vi "Polar Plot - Facade.vi"(0 "Data In":T3 {"phase (deg)" format="%0.2f"; "magnitude" format="%0.2f"}, 2 "Display State In":T1={"Plot Attributes"={"maximum"=2.0, "minimum"=0.0, "clip to min"=FALSE, "log"=FALSE, "grid color"=3381657, "plot color"=16711680, "fmt and prec"={"format"=enum."Decimal", "precision"=2}, "visible section"=4}, "Desired Font"=enum."Application Font", "User-Specified Font"={"Font Name:"="Arial", "Size"=9, "Strikeout?"=FALSE, "Italic?"=FALSE, "Underline?"=FALSE, "Outline?"=FALSE, "Shadow?"=FALSE, "Bold?"=FALSE}} {"Plot Attributes"."minimum" format="%0.2f"; "Plot Attributes"."maximum" format="%0.2f"}, 3 "Container State":T2) -> (6 "Data Out":T3 {"phase (deg)" format="%0.2f"; "magnitude" format="%0.2f"}, 7 "Display State Out":T1={"Plot Attributes"={"maximum"=2.0, "minimum"=0.0, "clip to min"=FALSE, "log"=FALSE, "grid color"=3381657, "plot color"=16711680, "fmt and prec"={"format"=enum."Decimal", "precision"=2}, "visible section"=4}, "Desired Font"=enum."Application Font", "User-Specified Font"={"Font Name:"="Arial", "Size"=9, "Strikeout?"=FALSE, "Italic?"=FALSE, "Underline?"=FALSE, "Outline?"=FALSE, "Shadow?"=FALSE, "Bold?"=FALSE}} {"Plot Attributes"."minimum" format="%0.2f"; "Plot Attributes"."maximum" format="%0.2f"}, 8 "Action":T4)   [LabVIEW 2009, in "Polar Plot.xctl"]
doc: "Demonstration of an XControl.\n\nAAL 9/09"
uses:
  Polar Plot.xctl
  <vilib>/_xctls/Action.ctl
  Polar Plot - Data.ctl
  <vilib>/_xctls/Container State.ctl
  Polar Plot - State.ctl
  <vilib>/_xctls/XControlSupport.lvlib
panel:
  out "Picture":picture
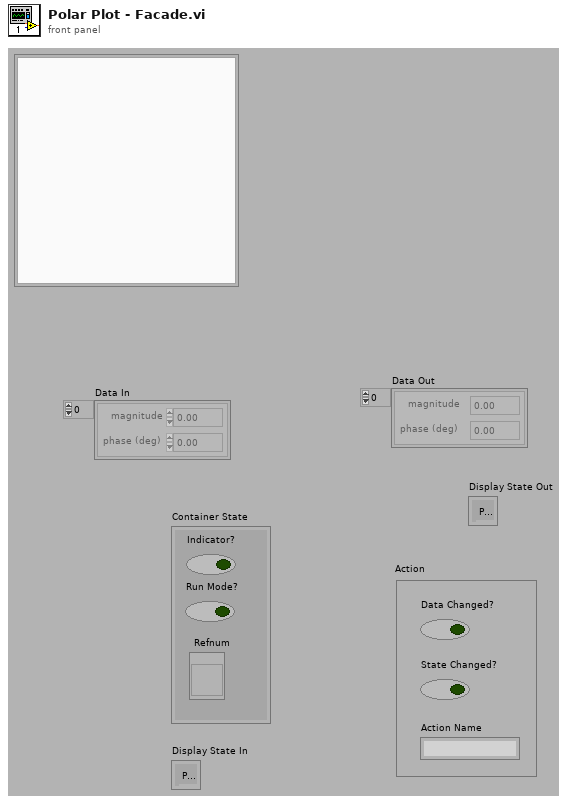
[diagram p1: front panel]
types:
  T1 = typedef "Polar Plot.xctl/Polar Plot - State.ctl" = cluster{"Plot Attributes":cluster{"maximum":dbl, "minimum":dbl, "clip to min":bool, "log":bool, "grid color":u32, "plot color":u32, "fmt and prec":cluster{"format":enum8{"Decimal", "Scientific", "Engineering", "Binary", "Octal", "Hex"}, "precision":u8}, "visible section":u16}, "Desired Font":enum16{"User-specified Font", "Application Font", "System Font", "Dialog Font"}, "User-Specified Font":cluster{"Font Name:":string, "Size":i16, "Strikeout?":bool, "Italic?":bool, "Underline?":bool, "Outline?":bool, "Shadow?":bool, "Bold?":bool}}
  T2 = typedef "XControlSupport.lvlib/Container State.ctl" = cluster{"Indicator?":bool, "Run Mode?":bool, " Refnum":refnum<vi>}
  T3 = typedef "Polar Plot.xctl/Polar Plot - Data.ctl" = cluster{"magnitude":dbl, "phase (deg)":dbl}[]
  T4 = typedef "XControlSupport.lvlib/Action.ctl" = cluster{"Data Changed?":bool, "State Changed?":bool, "Action Name":string}
  T5 = cluster{"Plot Attributes":cluster{"maximum":dbl, "minimum":dbl, "clip to min":bool, "log":bool, "grid color":u32, "plot color":u32, "fmt and prec":cluster{"format":enum8{"Decimal", "Scientific", "Engineering", "Binary", "Octal", "Hex"}, "precision":u8}, "visible section":u16}, "Desired Font":enum16{"User-specified Font", "Application Font", "System Font", "Dialog Font"}, "User-Specified Font":cluster{"Font Name:":string, "Size":i16, "Strikeout?":bool, "Italic?":bool, "Underline?":bool, "Outline?":bool, "Shadow?":bool, "Bold?":bool}}
  T6 = cluster{"Font Name:":string, "Size":i16, "Strikeout?":bool, "Italic?":bool, "Underline?":bool, "Outline?":bool, "Shadow?":bool, "Bold?":bool}
  T7 = enum16{"User-specified Font", "Application Font", "System Font", "Dialog Font"}
  T8 = cluster{"maximum":dbl, "minimum":dbl, "clip to min":bool, "log":bool, "grid color":u32, "plot color":u32, "fmt and prec":cluster{"format":enum8{"Decimal", "Scientific", "Engineering", "Binary", "Octal", "Hex"}, "precision":u8}, "visible section":u16}
  T9 = typedef "LVBoundsTypeDef.ctl" = cluster{"Width":u32, "Height":u32}
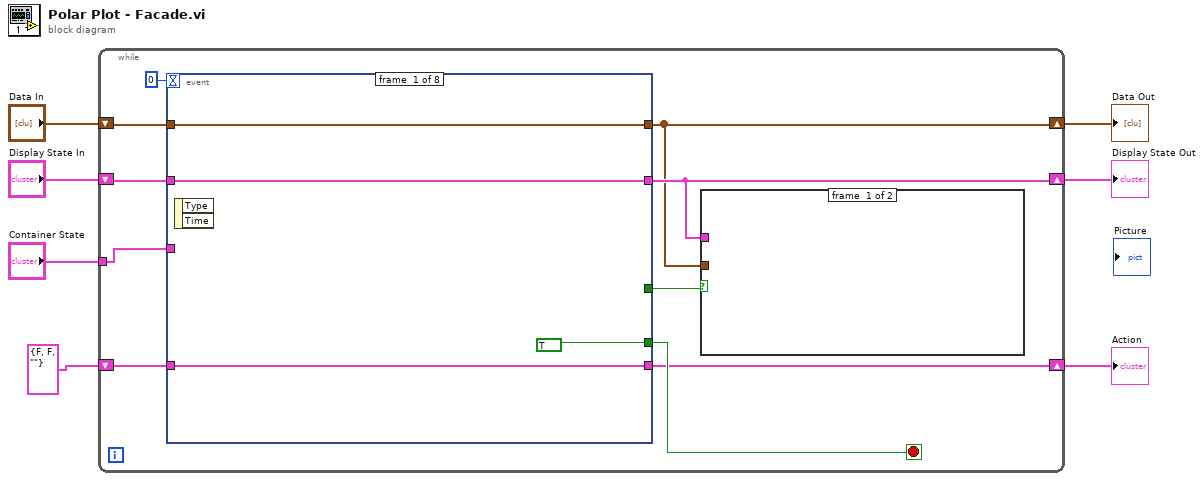
[diagram p0: block diagram]
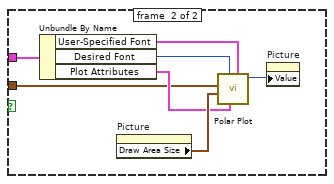
[diagram p2: hidden frame]
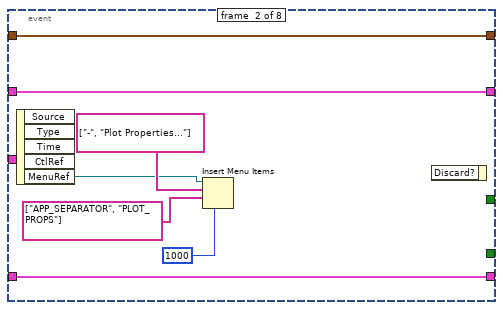
[diagram p3: hidden frame]
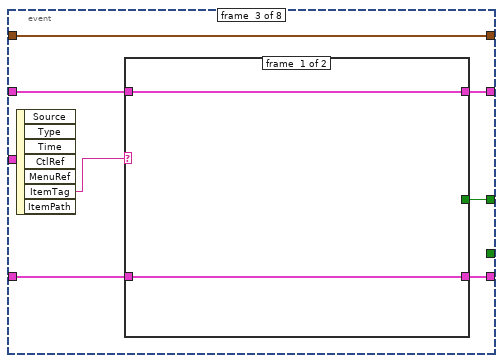
[diagram p4: hidden frame]
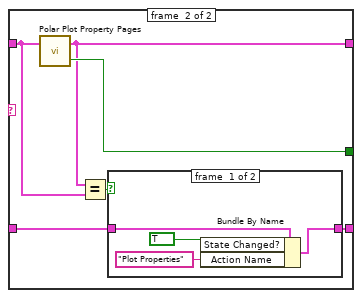
[diagram p5: hidden frame]
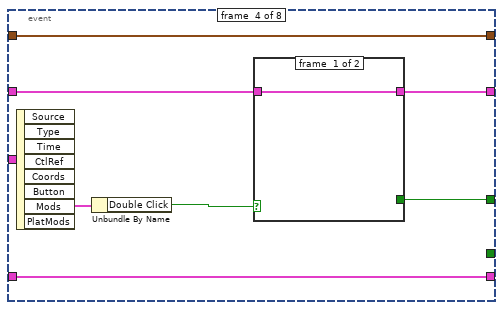
[diagram p7: hidden frame]
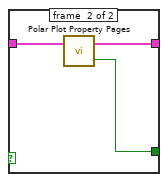
[diagram p8: hidden frame]
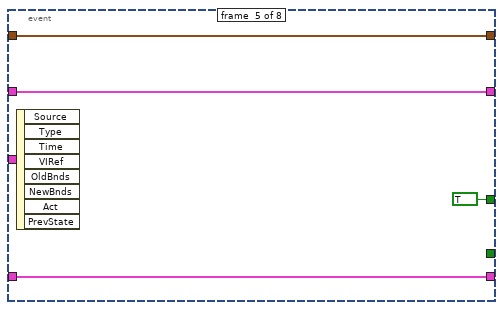
[diagram p9: hidden frame]
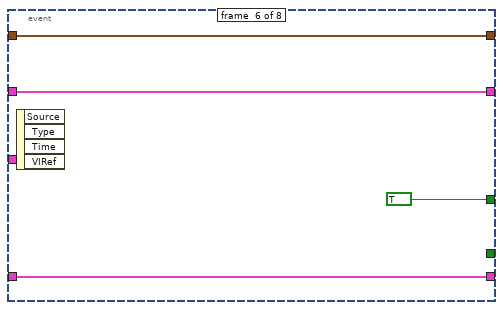
[diagram p10: hidden frame]
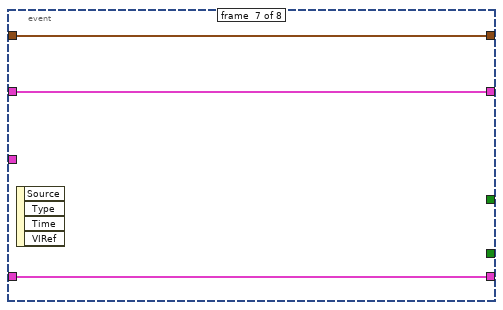
[diagram p11: hidden frame]
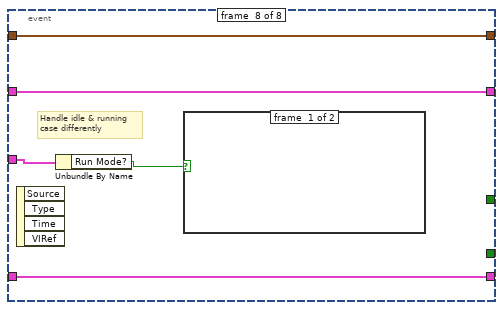
[diagram p12: hidden frame]
diagram:
  n1 = while {
    shift-right: [w9] -> w4
    shift-left: "Display State In" -> [w14]
    tunnel: "Container State" -> [w13]
    shift-right: [w8] -> w7
    shift-left: "Data In" -> [w15]
    shift-right: [w10] -> w1
    shift-left: T4 {"Data Changed?"=FALSE, "State Changed?"=FALSE, "Action Name"=""} ("Data Changed?") -> [w12]
    stop <- w11 stop-if-true
    n2 = event shown="[2] \"Picture\": Shortcut Menu Selection (User)" {
      selector: _ -> [_ _ _ _ _ _ _ _]
      dyn-events: _ -> [_ _ _ _ _ _ _ _]
      timeout: 0 -> [_ _ _ _ _ _ _ _]
      tunnel: w14 -> [w26 w32 w41 w62 w67 w73 w77 w80]
      tunnel: [w26 w32 w40 w61 w67 w73 w77 w80] -> w9
      tunnel: [TRUE _ _ _ _ _ _ _] -> w11
      tunnel: w13 -> [_ _ _ _ _ _ _ w81]
      tunnel: w15 -> [w25 w33 w38 w58 w68 w72 w76 w79]
      tunnel: [w25 w33 w38 w58 w68 w72 w76 w79] -> w8
      tunnel: [w27 w34 w37 w59 w69 w74 w75 w78] -> w10
      tunnel: w12 -> [w27 w34 w36 w59 w69 w74 w75 w78]
      tunnel: [_ _ w39 w60 TRUE ("OK?") TRUE _ _] -> w16
      event #0 {
        n3 = event-data() -> ()  [unwired: 1 in, 2 out]
      }
      event #1 {
        n4 = event-data() -> ("MenuRef"=w29:refnum<k9>)  [unwired: 1 in, 4 out]
        n5 = Insert Menu Items(4:1000, 7:string[] ["APP_SEPARATOR", "PLOT_PROPS"], 8:string[] ["-", "Plot Properties..."], 9:w29) -> ()  [unwired: 2 in, 3 out]
        n6 = event-data() -> ()  [unwired: 2 in, 1 out]
      }
      event #2 {
        n7 = event-data() -> ("ItemTag"=w42:string)  [unwired: 1 in, 6 out]
        n8 = case shown="\"PLOT_PROPS\"" w42 {
          tunnel: w41 -> [w44 w49]
          tunnel: [w44 w48] -> w40
          tunnel: [_ w50] -> w39
          tunnel: [w43 w46] -> w37
          tunnel: w36 -> [w43 w45]
          frame #0 {
          }
          frame #1 {
            n9 = call "Polar Plot Property Pages.vi"("Display State In"=w49) -> ("OK?"=w50:bool, "Display State Out"=w48:T5)  [unwired: 1 in]
            n10 = Equal?(x=w48, y=w49) -> (x = y?=w47:bool)
            n11 = case shown="False" w47 {
              tunnel: [w54 w55] -> w46
              tunnel: w45 -> [w53 w55]
              frame #0 {
                n12 = Bundle By Name(cluster=w53, "State Changed?"=TRUE, "Action Name"="Plot Properties") -> (w54:T4)
              }
              frame #1 {
              }
            }
          }
        }
      }
      event #3 {
        n13 = event-data() -> ("Mods"=w57:cluster{"Double Click":bool, "Menu Key":bool})  [unwired: 1 in, 7 out]
        n14 = Unbundle By Name(w57) -> ("Double Click"=w56:bool)
        n15 = case shown="True" w56 {
          tunnel: w62 -> [w63 w66]
          tunnel: [w63 w65] -> w61
          tunnel: [_ w64] -> w60
          frame #0 {
          }
          frame #1 {
            n16 = call "Polar Plot Property Pages.vi"("Display State In"=w66) -> ("OK?"=w64:bool, "Display State Out"=w65:T5)  [unwired: 1 in]
          }
        }
      }
      event #4 {
        n17 = event-data() -> ()  [unwired: 1 in, 8 out]
      }
      event #5 {
        n18 = event-data() -> ()  [unwired: 1 in, 4 out]
      }
      event #6 {
        n19 = event-data() -> ()  [unwired: 1 in, 4 out]
      }
      event #7 {
        # "Handle idle & running\ncase differently"
        n20 = event-data() -> ()  [unwired: 1 in, 4 out]
        n21 = Unbundle By Name(w81) -> ("Run Mode?"=w82:bool)
        n22 = case shown="False" w82 {
          frame #0 {
          }
          frame #1 {
          }
        }
      }
    }
    n23 = case shown="True" w16 {
      tunnel: w9 -> [_ w21]
      tunnel: w8 -> [_ w19]
      frame #0 {
      }
      frame #1 {
        n24 = Unbundle By Name(w21) -> ("User-Specified Font"=w20:T6, "Desired Font"=w23:T7, "Plot Attributes"=w22:T8)
        n25 = property on="Picture" class="Pict"() -> ("Draw Area Size"=w24:T9)  [unwired: 2 in, 2 out]
        n26 = call <vilib>:"Polar Plot.vi"("[user-specified font]"=w20, "polar attributes"=w22, "desired font(Application)"=w23, "dimensions (w,h)"=w24, "data array [mag, phase (deg)]"=w19) -> ("new picture"=w18:picture)  [unwired: 6 in]
        n27 = property on="Picture" class="Pict"("Value"=w18) -> ()  [unwired: 2 in, 2 out]
      }
    }
  }
  "Display State Out" <- w4
  "Data Out" <- w7
  "Action" <- w1
